vi "CheckLic - 副本.vi"(0 "路径":path, 2 "对外文件夹名称":string) -> (6 "鉴权通过":bool)   [LabVIEW 2013]
panel:
  out "错误输出":errorcluster
  in  "簇":T1
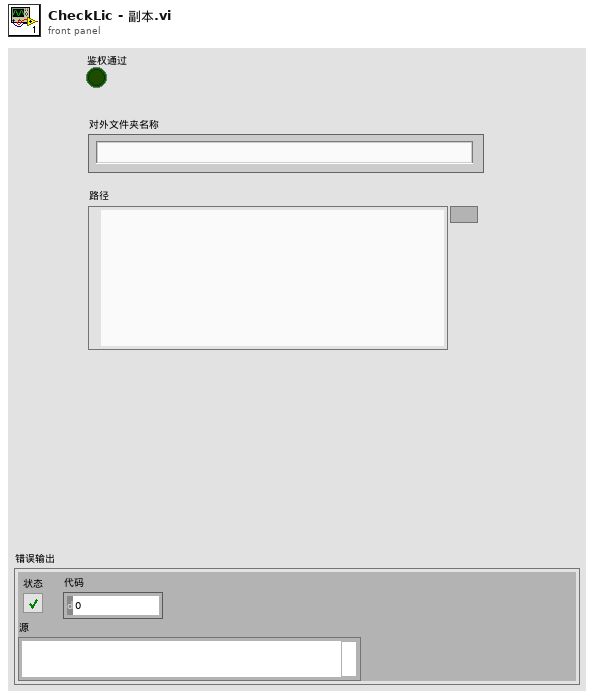
[diagram p1: front panel]
types:
  T1 = cluster{"RandomCode":string, "LicCode":string, "Times":dbl, "StartTime":string, "EndTime":string, "参数配置":bool, "参数生成":bool, "强制操作":bool, "数据保存":bool}
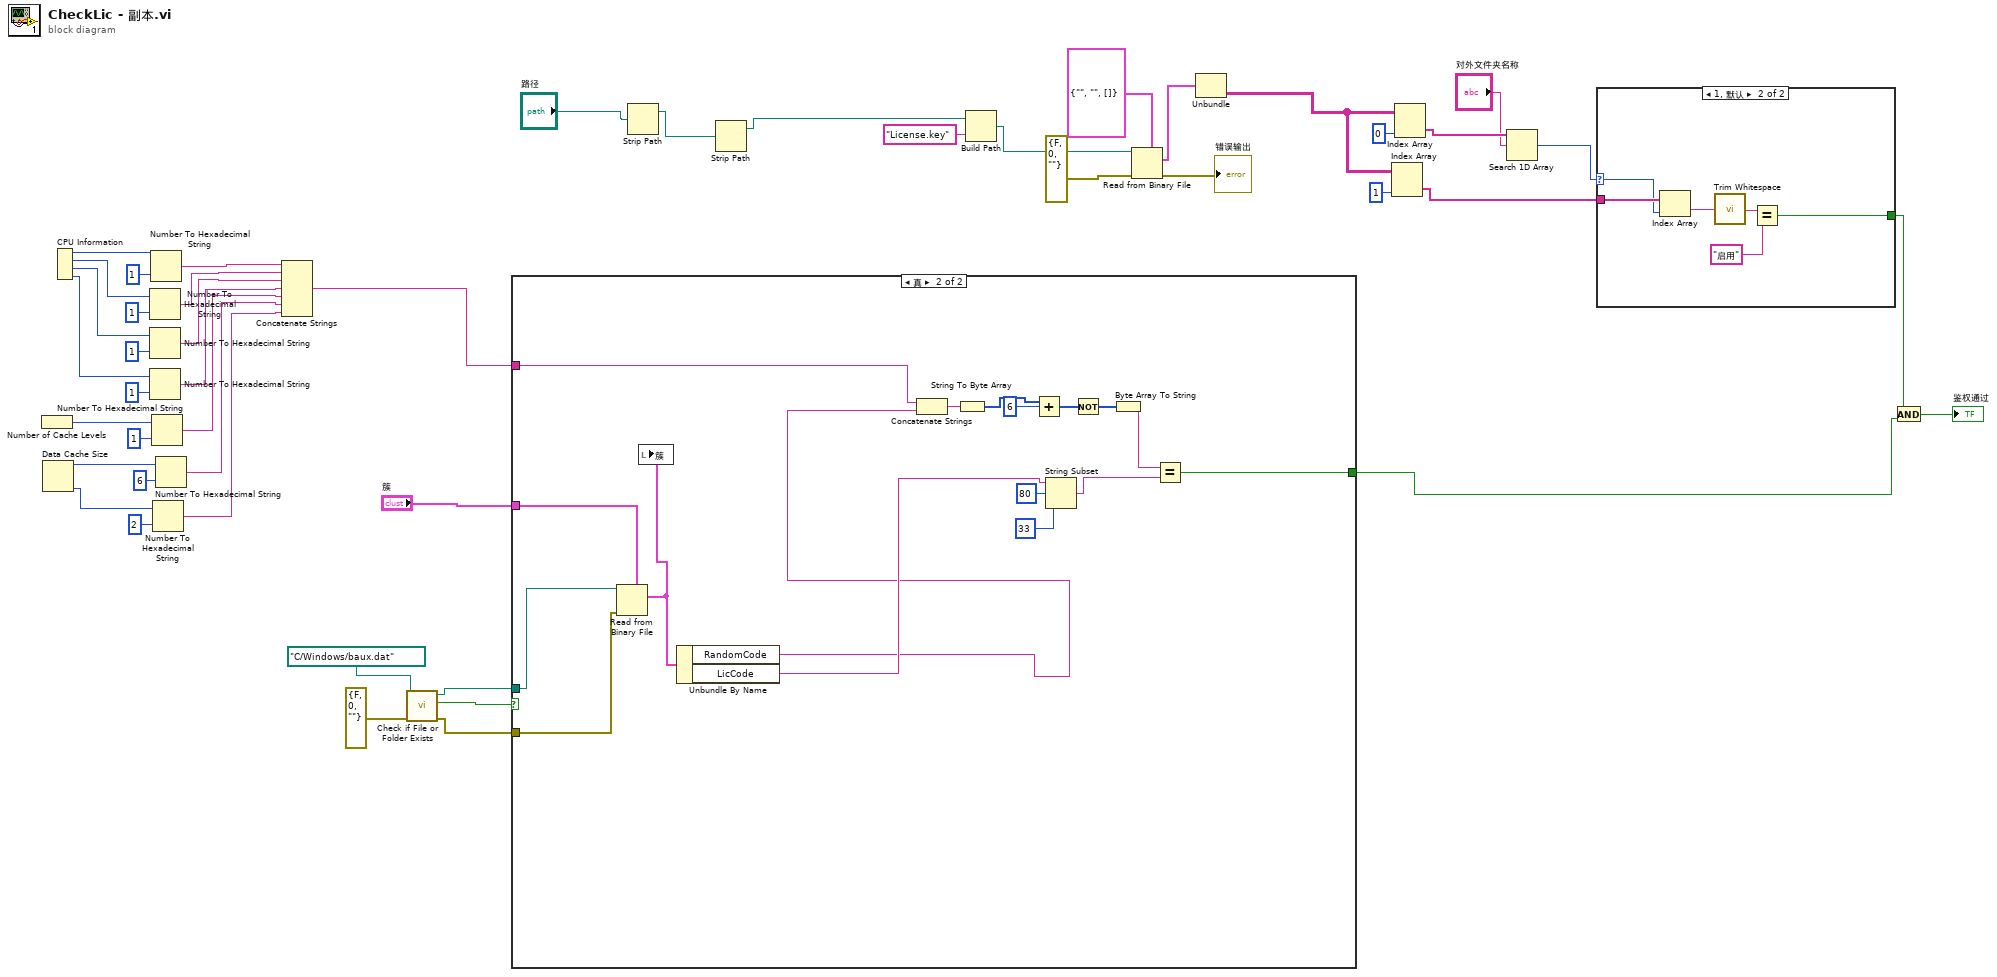
[diagram p0: block diagram]
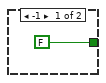
[diagram p2: hidden frame]
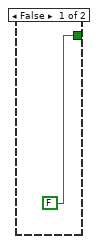
[diagram p3: hidden frame]
diagram:
  n1 = Number of Cache Levels() -> (w32:i32)
  n2 = Data Cache Size() -> (4:w33:i32, 7:w35:i32)  [unwired: 1 in]
  n3 = CPU Information() -> (4:w23:i32, 5:w27:i32, 6:w28:i32, 7:w29:i32)
  n4 = Number To Hexadecimal String(1:i16 1 ("宽度(-)"), 2:w27) -> (0:w37:string)
  n5 = Number To Hexadecimal String(1:i16 1 ("宽度(-)"), 2:w28) -> (0:w38:string)
  n6 = Number To Hexadecimal String(1:i16 1 ("宽度(-)"), 2:w29) -> (0:w39:string)
  n7 = Number To Hexadecimal String(1:i16 1 ("宽度(-)"), 2:w23) -> (0:w36:string)
  n8 = Number To Hexadecimal String(1:i16 1 ("宽度(-)"), 2:w32) -> (0:w40:string)
  n9 = Number To Hexadecimal String(1:i16 2 ("宽度(-)"), 2:w35) -> (0:w42:string)
  n10 = Number To Hexadecimal String(1:i16 6 ("宽度(-)"), 2:w33) -> (0:w41:string)
  n11 = Concatenate Strings(w36, w37, w38, w39, w40, w41, w42) -> (w21:string)
  n12 = call <vilib>:"Check if File or Folder Exists.vi"("error in (no error)"=errorcluster {"status"=FALSE, "code"=0, "source"=""}, "path"=path "C:/Windows/baux.dat" ("文件（使用对话框）")) -> ("error out"=w20:errorcluster, "file or folder exists?"=w45:bool, "dup path"=w44:path)  [unwired: 7 in]
  n13 = case shown="真" w45 {
    tunnel: w44 -> [_ w54]
    tunnel: "簇" -> [_ w64]
    tunnel: w21 -> [_ w61]
    tunnel: [FALSE w50] -> w5
    tunnel: w20 -> [_ w51]
    frame False {
    }
    frame True {
      n14 = Read from Binary File(5:w64, 8:w51, 11:w54) -> (2:w53:T1)  [unwired: 3 in, 3 out]
      n15 = local write "簇"(w53) -> ()
      n16 = Unbundle By Name(w53) -> ("RandomCode"=w49:string, "LicCode"=w52:string)
      n17 = Concatenate Strings(w61, w49) -> (w55:string)
      n18 = String To Byte Array(string=w55) -> (unsigned byte array=w60:u8[])
      n19 = Add(x=w60, y=u8 6) -> (x+y=w58:u8[])
      n20 = String Subset(string=w52, offset (0)=80 ("偏移量(0)"), length (rest)=33 ("长度（剩余）")) -> (substring=w57:string)
      n21 = Not(x=w58) -> ()  [unwired: 1 out]
      n22 = Byte Array To String(unsigned byte array=w58) -> (string=w56:string)
      n23 = Equal?(x=w56, y=w57) -> (x = y?=w50:bool)
    }
  }
  n24 = Strip Path(path="路径") -> (stripped path=w2:path)  [unwired: 1 out]
  n25 = Strip Path(path=w2) -> (stripped path=w1:path)  [unwired: 1 out]
  n26 = Build Path(base path=w1, name or relative path="License.key" ("名称或相对路径")) -> (appended path=w18:path)
  n27 = Read from Binary File(5:cluster{string, string, "ItemNames":string[][]} {"", "", "ItemNames"=[]} ("输出簇"), 8:errorcluster {"status"=FALSE, "code"=0, "source"=""} ("错误输入"), 11:w18) -> (0:→"错误输出":errorcluster, 2:w15:cluster{string, string, "ItemNames":string[][]})  [unwired: 3 in, 2 out]
  n28 = Unbundle(w15) -> ("ItemNames"=w8:string[][])  [unwired: 2 out]
  n29 = Index Array(array=w8, index (col)=1 ("禁用的索引 (列)")) -> (element=w7:string[])  [unwired: 1 in]
  n30 = Index Array(array=w8, index (col)=0 ("禁用的索引 (列)")) -> (element=w12:string[])  [unwired: 1 in]
  n31 = Search 1D Array(1D array=w12, element="对外文件夹名称") -> (index of element=w10:i32)  [unwired: 1 in]
  n32 = case shown="1, 默认" w10 {
    selector: w10 -> [_ w70]
    tunnel: w7 -> [_ w71]
    tunnel: [FALSE ("status") w66] -> w6
    frame -1 {
    }
    frame 1, Default {
      n33 = Index Array(array=w71, index=w70) -> (element=w69:string)
      n34 = call <vilib>:"Trim Whitespace.vi"("string"=w69) -> ("trimmed string"=w68:string)  [unwired: 1 in]
      n35 = Equal?(x=w68, y="启用") -> (x = y?=w66:bool)
    }
  }
  n36 = And(x=w6, y=w5) -> (x .and. y?=→"鉴权通过":bool)
